vi "Navigate and Wait.vi"(6 "Timeout (Inf)":i32=-1, 7 "html Source (URL)":bool, 8 "error in (no error)":errorcluster, 10 "Source":string, 11 "WebView2 Control in":refnum<class "WebView2 Control.lvclass">) -> (0 "error out":errorcluster, 2 "Timed Out":bool, 3 "WebView2 Control out":refnum<class "WebView2 Control.lvclass">)   [LabVIEW 2020, in "WebView2.lvlib" / "WebView2 Control.lvclass"]
uses:
  WebView2 Control.lvclass
  C:/Users/Simon/Documents/GitHub/LV-WebView2/Source/Libs/Microsoft.Web.WebView2.Core.dll
  Libs/Microsoft.Web.WebView2.Core.dll
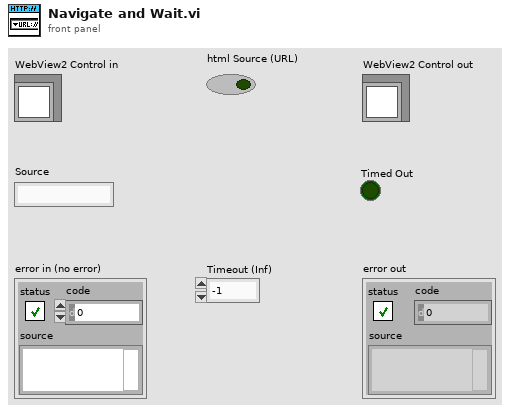
[diagram p1: front panel]
types:
  T1 = typedef "WebView2.lvlib/WebView2 Control.lvclass/Events.ctl" = cluster{"Navigation Complete Event":refnum<user-event>, "Source Changed Event":refnum<user-event>, "Document Title Changed Event":refnum<user-event>, "Status Bar Text Changed":refnum<user-event>, "Web Message Received":refnum<user-event>, "Window Close Requested":refnum<user-event>, "DOM Loaded":refnum<user-event>, "Navigation Started Event":refnum<user-event>}
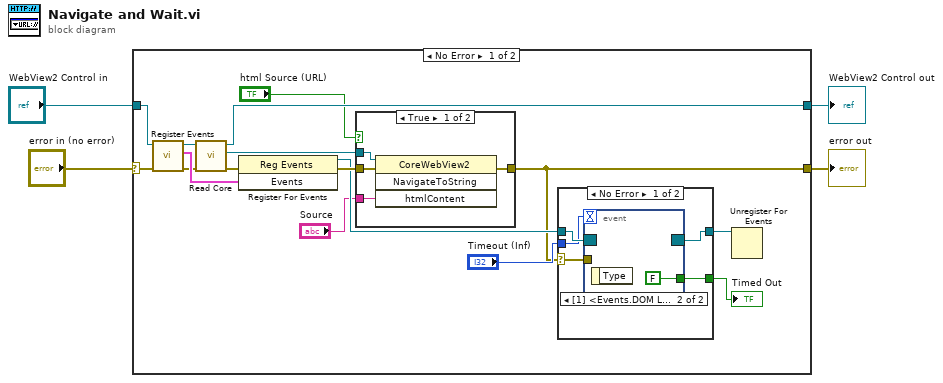
[diagram p0: block diagram]
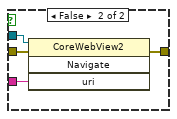
[diagram p2: hidden frame]
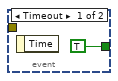
[diagram p3: hidden frame]
diagram:
  n1 = case shown="No Error" "error in (no error)" {
    selector: "error in (no error)" -> [w11 w37]
    tunnel: "WebView2 Control in" -> [w5 w38]
    tunnel: [w9 w38] -> w2
    tunnel: [w13 w37] -> w1
    frame No Error {
      n2 = call "Register Events.vi"("error in (no error)"=w11, "WebView2 Control in"=w5) -> ("error out"=w8:errorcluster, "Events"=w17:T1, "WebView2 Control out"=w10:refnum<class "WebView2 Control.lvclass">)  [unwired: 7 in]
      n3 = call "Read Core.vi"("error in (no error)"=w8, "WebView2.lvlib:WebView2 Control.lvclass"=w10) -> ("error out"=w7:errorcluster, "Webview2 Core"=w12:refnum<k24>, "WebView2.lvlib:WebView2 Control.lvclass"=w9:refnum<class "WebView2 Control.lvclass">)  [unwired: 7 in]
      n4 = register-events(error in=w7, w17) -> (reference out=w19:refnum<event-registration>, error out=w20:errorcluster)  [unwired: 1 in]
      n5 = case shown="True" "html Source (URL)" {
        tunnel: w20 -> [w24 w28]
        tunnel: "Source" -> [w23 w27]
        tunnel: [w22 w26] -> w13
        tunnel: w12 -> [w21 w25]
        frame True {
          n6 = invoke class="CoreWebView2" method="NavigateToString"(reference=w21, error in=w24, "htmlContent"=w23) -> (error out=w22:errorcluster)  [unwired: 1 in, 3 out]
        }
        frame False {
          n7 = invoke class="CoreWebView2" method="Navigate"(reference=w25, error in=w28, "uri"=w27) -> (error out=w26:errorcluster)  [unwired: 1 in, 3 out]
        }
      }
      n8 = case shown="No Error" w13 {
        selector: w13 -> [w29 _]
        tunnel: w19 -> [w33 w36]
        tunnel: [w32 _] -> w18
        tunnel: "Timeout (Inf)" -> [w31 _]
        tunnel: [w30 w36] -> w14
        frame No Error {
          n9 = event shown="[1] <Events.DOM Loaded>: User Event" {
            selector: w33 -> [_ _]
            dyn-events: [_ _] -> w30
            timeout: w31 -> [_ _]
            tunnel: [TRUE FALSE] -> w32
            tunnel: w29 -> [_ _]
            event Timeout {
              n10 = event-data() -> ()  [unwired: 1 in, 1 out]
            }
            event User Event {
              n11 = event-data() -> ()  [unwired: 1 in, 1 out]
            }
          }
        }
        frame Error {
        }
      }
      "Timed Out" <- w18
      n12 = Unregister For Events(event registration refnum=w14) -> ()  [unwired: 1 in, 1 out]
    }
    frame Error {
    }
  }
  "error out" <- w1
  "WebView2 Control out" <- w2
